vi "Pos_Calculate location.vi"(5 "Front Panel.PanelBounds":T5, 7 "Origin":T1, 8 "Error":errorcluster, 9 "Point":T4, 11 "Vi To Move Settings":T2) -> (0 "Error Out":errorcluster, 3 "Vi To Move Settings Out":T2)   [LabVIEW 2020]
uses:
  <vilib>/Utility/miscctls.llb/LVRectTypeDef.ctl
  TypeDefs_Utility/Cluster_Top Left position.ctl
  TypeDefs_Utility/Cluster_FP on Point Set.ctl
  TypeDefs_Utility/ENUM RB_Pos_Quadrant Position.ctl
  <vilib>/Utility/miscctls.llb/LVPointTypeDef.ctl
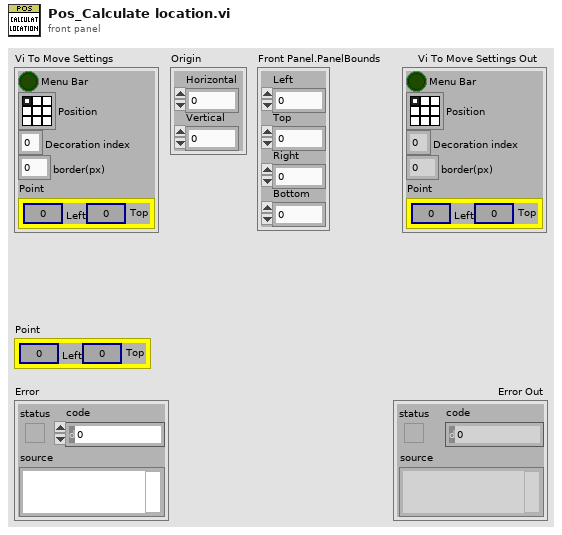
[diagram p1: front panel]
types:
  T1 = typedef "LVPointTypeDef.ctl" = cluster{"Horizontal":i16, "Vertical":i16}
  T2 = typedef "Cluster_FP on Point Set.ctl" = cluster{"Menu Bar":bool, "Position":T3, "Decoration index":i32, "border(px)":i32, "Point":T4}
  T3 = typedef "ENUM RB_Pos_Quadrant Position.ctl" = enum32{"LFT-TOP", "MID-TOP", "RGT-TOP", "LFT-CTR", "MID-CTR", "RGT-CTR", "LFT-BOT", "MID-BOT", "RGT-BOT"}
  T4 = typedef "Cluster_Top Left position.ctl" = cluster{"Left":i32, "Top":i32}
  T5 = typedef "LVRectTypeDef.ctl" = cluster{"Left":i16, "Top":i16, "Right":i16, "Bottom":i16}
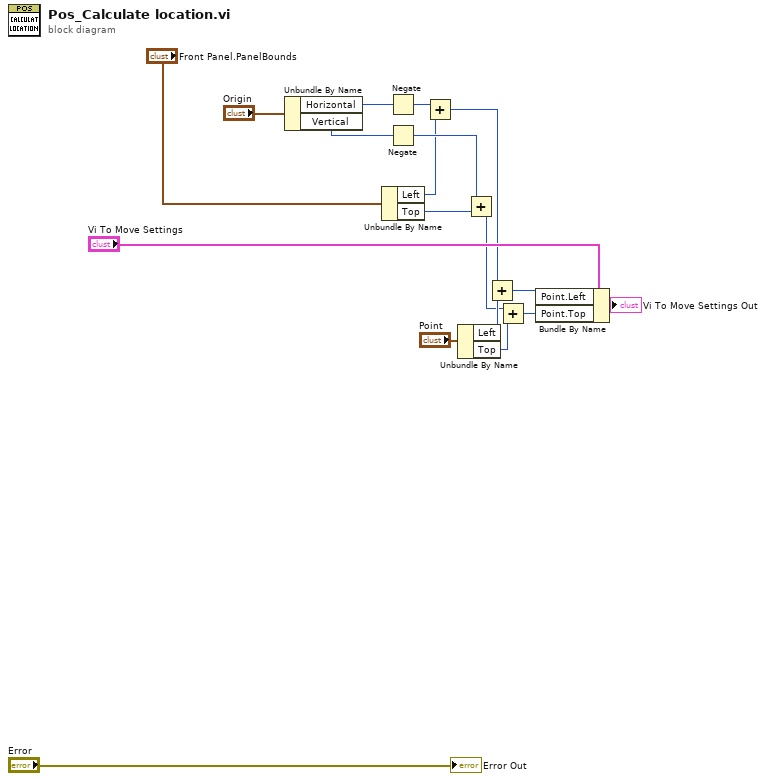
[diagram p0: block diagram]
diagram:
  n1 = Unbundle By Name("Origin") -> ("Horizontal"=w3:i16, "Vertical"=w4:i16)
  n2 = Unbundle By Name("Front Panel.PanelBounds") -> ("Left"=w5:i16, "Top"=w8:i16)
  n3 = Negate(x=w3) -> (-x=w6:i16)
  n4 = Negate(x=w4) -> (-x=w7:i16)
  n5 = Add(x=w6, y=w5) -> (x+y=w10:i16)
  n6 = Unbundle By Name("Point") -> ("Left"=w17:i32, "Top"=w16:i32)
  n7 = Add(x=w7, y=w8) -> (x+y=w9:i16)
  n8 = Add(x=w10, y=w17) -> (x+y=w11:i32)
  n9 = Add(x=w9, y=w16) -> (x+y=w12:i32)
  n10 = Bundle By Name(cluster="Vi To Move Settings", "Point.Left"=w11, "Point.Top"=w12) -> (→"Vi To Move Settings Out":T2)
  "Error Out" <- "Error"
